vi "Create.vi"(5 "Error In":refnum<class "Error.lvclass">, 8 "error in (no error)":errorcluster) -> (0 "error out":errorcluster, 3 "Error":refnum<class "Error.lvclass">)   [LabVIEW 2017, in "Transparent Assertions.lvlib" / "Constraints.lvlib" / "Error.lvclass"]
uses:
  Error.lvclass
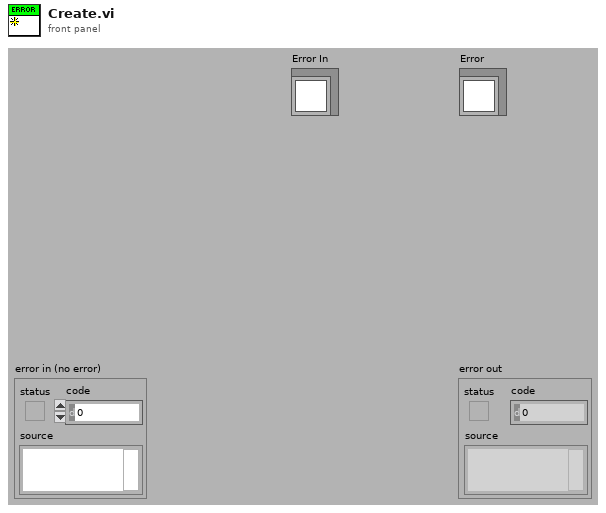
[diagram p1: front panel]
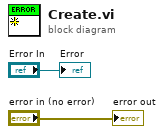
[diagram p0: block diagram]
diagram:
  "error out" <- "error in (no error)"
  "Error" <- "Error In"
